vi "slow_control_alpha_01.vi"() -> ()   [LabVIEW 2018]
uses:
  <instrlib>/Lake Shore 335/Lake Shore 335.lvlib
  <instrlib>/CAEN PSM/CAEN PSM.lvlib
panel:
  in  "stop":bool
  out "Anode resets in":string
  out "Voltages":dbl[](array[numeric])
  out "Started up?":bool
  out "Try 2 Inside loop":dbl[][](array[numeric])
  in  "Read T every N cycles":i32=2
  out "Time until next cycle":dbl
  in  "Time per cycle (s)":i32=2 caption="Time Target (s)"
  in  "input cluster":errorcluster
  in  "Allows tabs on \nfront panel":T1(tab)
  in  "Heater range":u16(ring) items=["Off", "Low (On)", "Medium", "High"]
  in  "Setpoint (°C)":dbl=-100.0
  in  "PID settings":T2
  in  "COM-port NI-box":refnum<visa-resource-name>
  in  "COM-port LakeShore":refnum<visa-resource-name>
  in  "ID Query":bool=TRUE
  in  "COM-port CAEN 1":refnum<visa-resource-name>
  in  "COM-port CAEN 2":refnum<visa-resource-name>
  in  "Sensor 2 Offset":dbl=1.0 format="%#_13g"
  in  "Sensor 2 Mult. Factor":dbl=25.0 format="%#_13g"
  in  "Sensor 1 Offset":dbl=0.44736 format="%#_13g"
  in  "Sensor 1 Mult. Factor":dbl=25.0 format="%#_13g"
  in  "Sensor 3 Offset":dbl=1.0 format="%#_13g"
  in  "Sensor 3 Mult. Factor":dbl=50.0 format="%#_13g"
  in  "Sensor 4 Offset":dbl=1.0 format="%#_13g"
  in  "Sensor 4 Mult. Factor":dbl=10.0 format="%#_13g"
  in  "Ignore Initialization Errors":bool caption="Ignore init. errors?"
  out "LakeShore status":bool
  out "NI-box status":bool
  out "CAEN 1 status":bool
  out "CAEN 2 status":bool
  out "Initialization status":bool
  in  "VSet (V)":dbl[](array[numeric])
  in  "IMax (uA)":dbl[](array[numeric])
  in  "VMax (V)":dbl[](array[numeric])
  out "Cathode":dbl(knob) scale=0.0..5000.0
  out "Anode":dbl(knob) scale=0.0..4000.0
  out "PMT 2":dbl(knob) scale=0.0..1000.0
  out "PMT 1":dbl(knob) scale=1.0..1000.0
  out "Vmon (V)":dbl[](array[numeric])
  out "IMon (uA)":dbl[](array[numeric])
  in  "Reset anode":bool
  in  "Kill every Y minutes":i32=10
  in  "Keep off for X seconds":i32=10
  out "Total cycles in Anode Reset Routine":i32
  out "Current modulated cycle number":i32
  out "VSet killed":bool
  out "VSet applied":bool
  out "Read V = 0":i32
  out "Error caen 1":errorcluster
  out "Error caen 2":errorcluster
  in  "Read V every N cycles":i16=120
  # "<- Proof of concept for New/Old T + New P"
  # "PMT 1"
  # "PMT 2"
  # "Anode"
  # "Cathode"
  # "Top gate"
  # "Bottom gate"
  # "seconds"
  # "Pressure correction settings"
  # "Connection settings"
  # "Lakeshore settings"
  # "Gain (P) (XX.X)"
  # "Reset (I) (XX.X)"
  # "Rate (D) (X.X%)"
  # "Pressure correction factors go here.\nPrecisely, offsets and multiplication factors\nin the voltages passed from the pressure-\nsensors to the NI-box."
  # "<- Change wiring"
  # "Might need to split up NI-box com port.\nPreferable to task it with measuring T\nand P seperately.\nPerhaps need to set task per single channel."
  # "Alarm indicators"
  # "CAEN 1"
  # "Data"
  # "PMT 1"
  # "PMT 1"
  # "PMT 2"
  # "PMT 2"
  # "Anode"
  # "Anode"
  # "Cathode"
  # "Cathode"
  # "Arrays from CAEN 2 go here"
  # "Top gate"
  # "Top gate"
  # "Bottom gate"
  # "Bottom gate"
  # "Settings"
  # "PMT 1"
  # "PMT 1"
  # "PMT 2"
  # "PMT 2"
  # "Anode"
  # "Anode"
  # "Cathode"
  # "Cathode"
  # "CAEN 2"
  # "Top gate"
  # "Top gate"
  # "Bottom gate"
  # "Bottom gate"
  # "PMT 1"
  # "PMT 2"
  # "Anode"
  # "Cathode"
  # "Needle gauges or other displays go here"
  # "Top gate"
  # "Bottom gate"
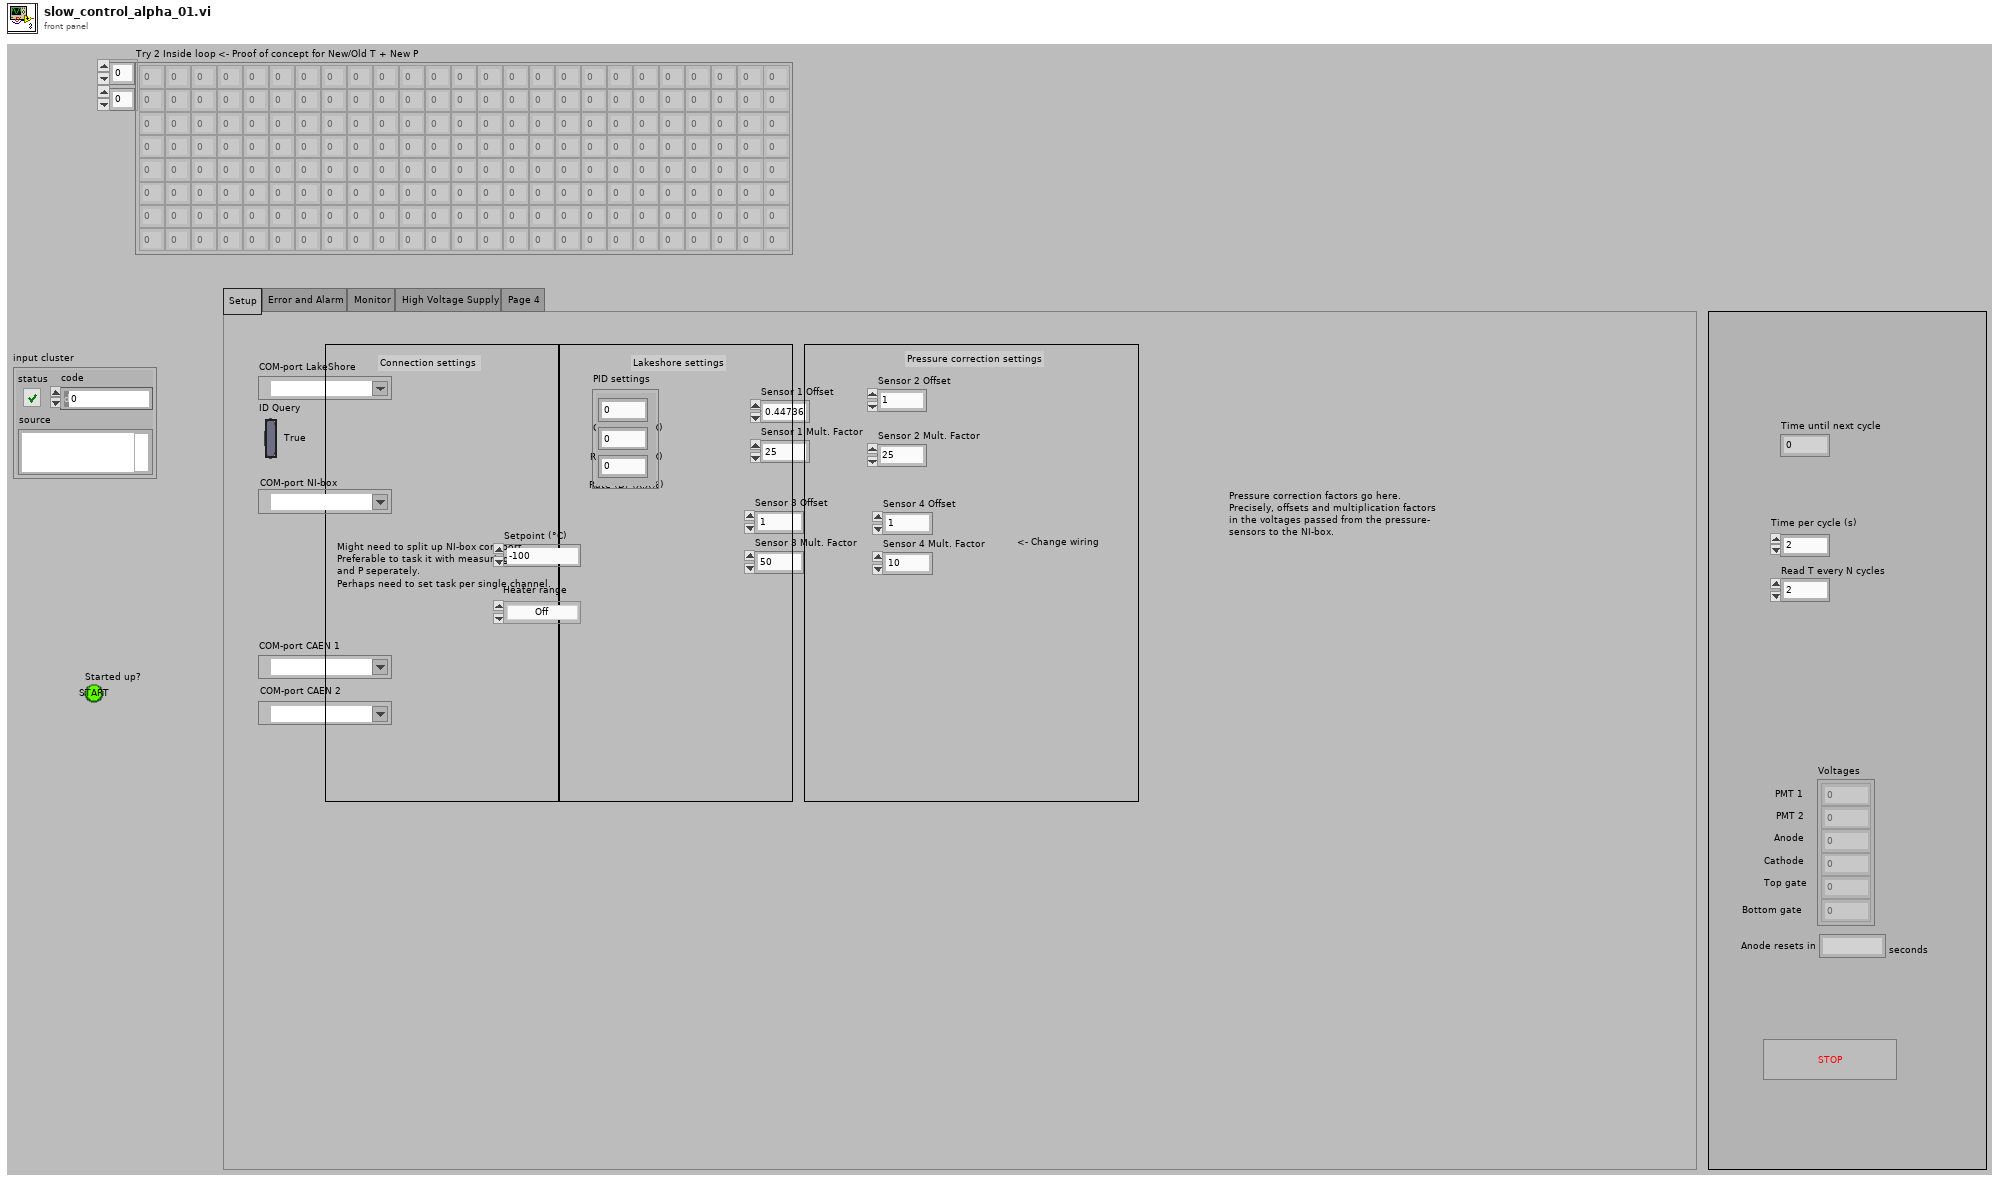
[diagram p1: front panel]
types:
  T1 = enum32{"Setup", "Error and Alarm", "Monitor", "High Voltage Supply", "Page 4"}
  T2 = cluster{"Numeric":dbl, "Numeric 2":dbl, "Numeric 3":dbl}
  T3 = cluster{"Flow Control":u16, "Stop Bits":u16, "Data Bits":u16, "Parity":u16, "Baud Rate":u32}
  T4 = cluster{"VISA resource name out":refnum<visa-resource-name>, "error out":errorcluster}
  T5 = cluster{"VMax (V)":dbl[], "IMax (uA)":dbl[], "VSet (V)":dbl[]}
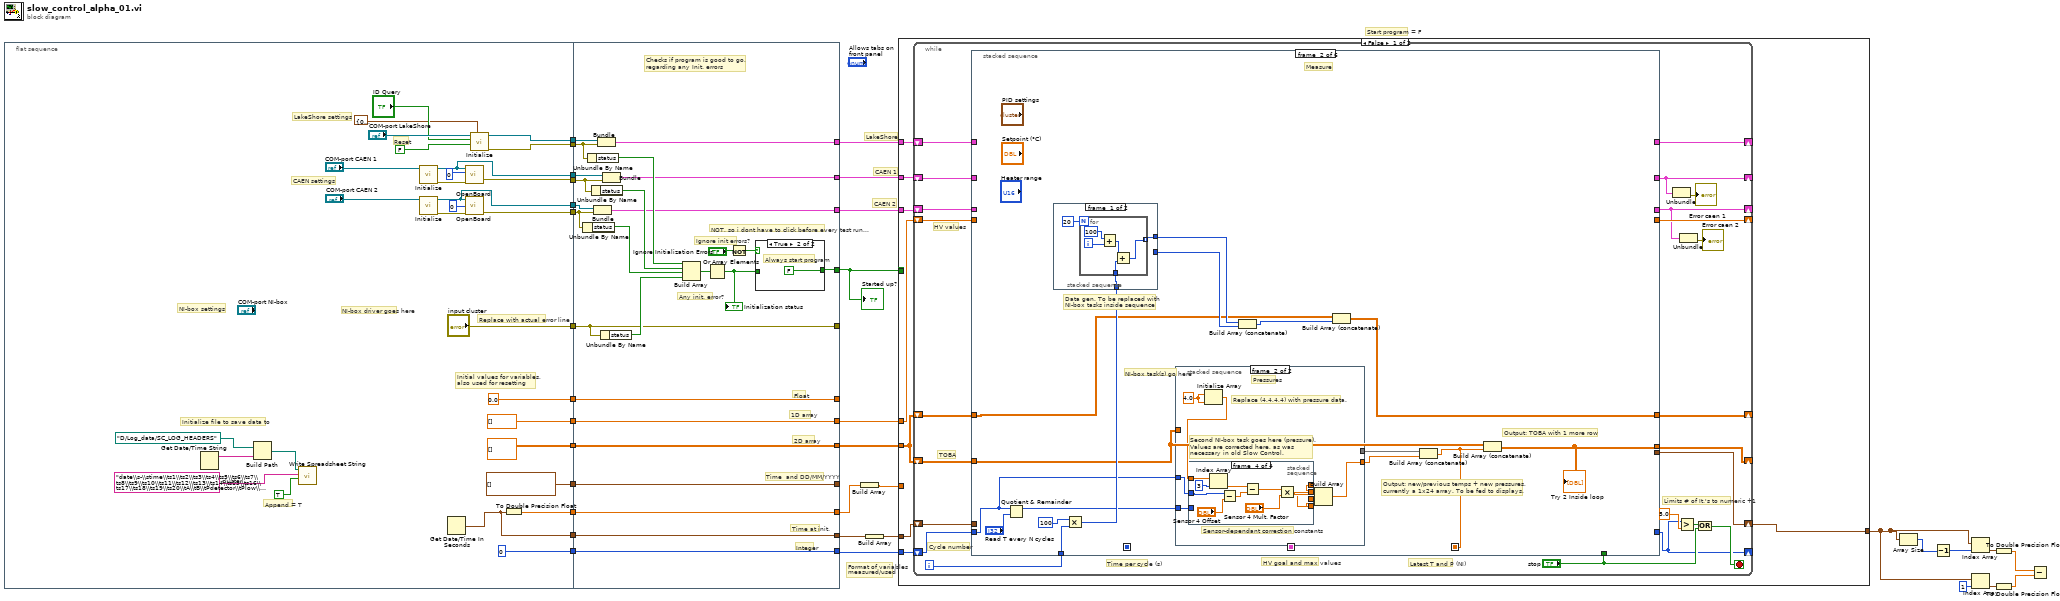
[diagram p0: block diagram]
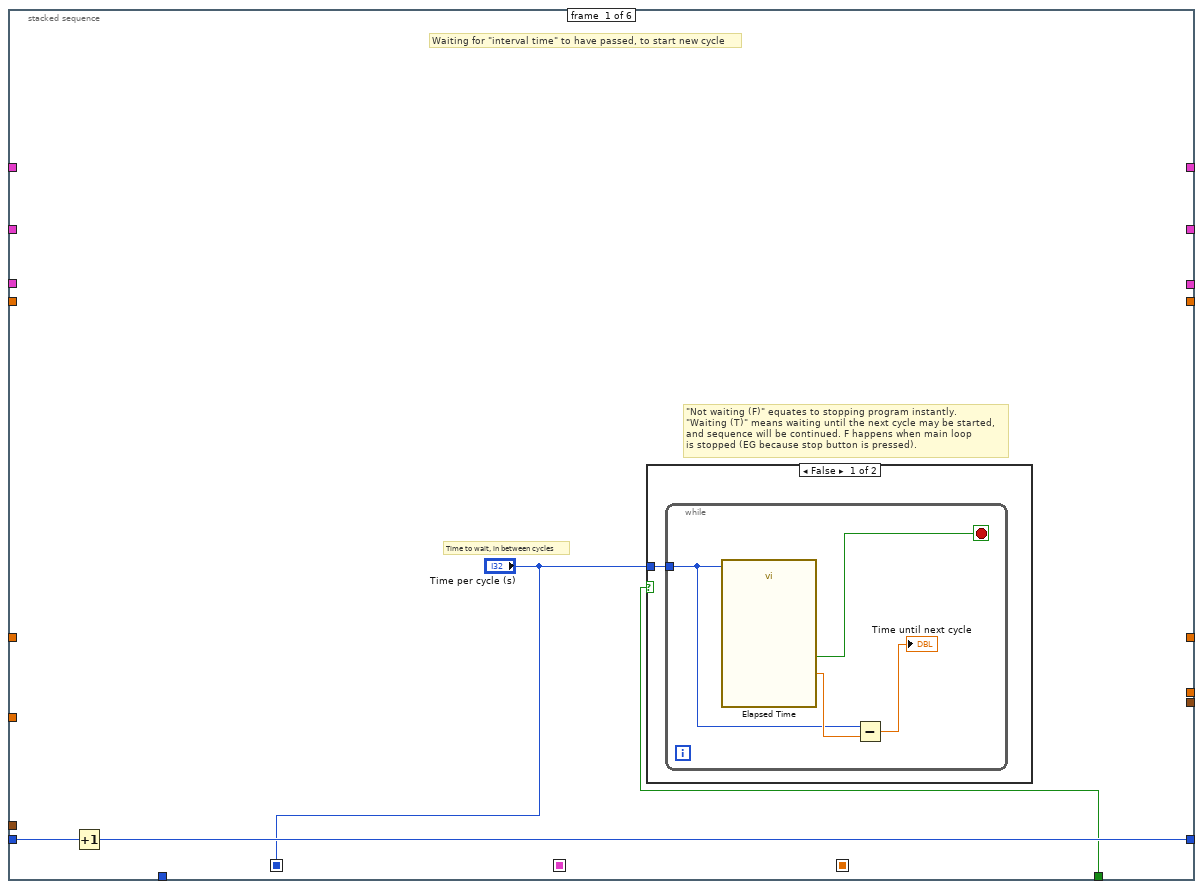
[diagram p2: hidden frame]
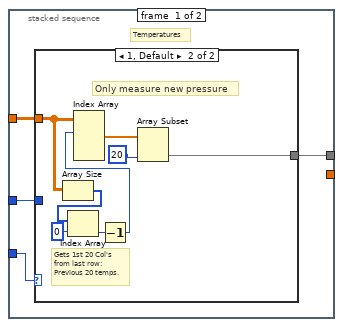
[diagram p4: hidden frame]
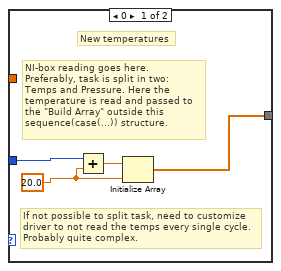
[diagram p5: hidden frame]
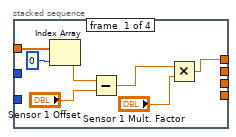
[diagram p6: hidden frame]
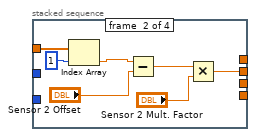
[diagram p7: hidden frame]
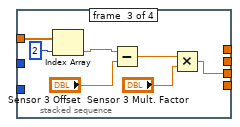
[diagram p8: hidden frame]
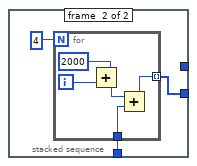
[diagram p9: hidden frame]
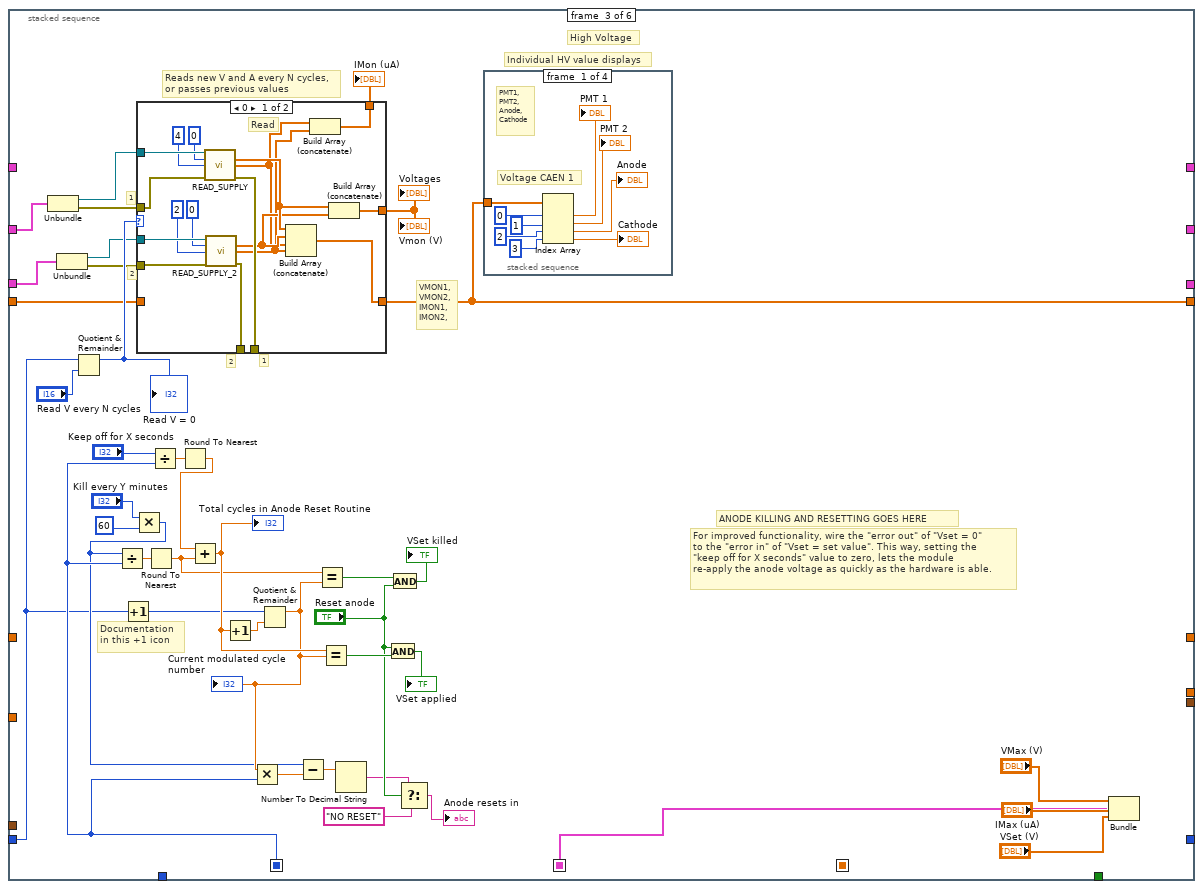
[diagram p10: hidden frame]
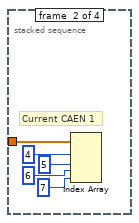
[diagram p11: hidden frame]
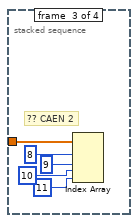
[diagram p12: hidden frame]
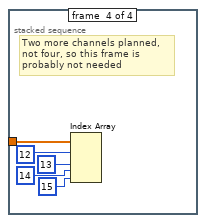
[diagram p13: hidden frame]
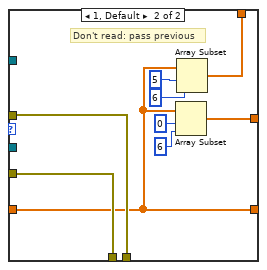
[diagram p14: hidden frame]
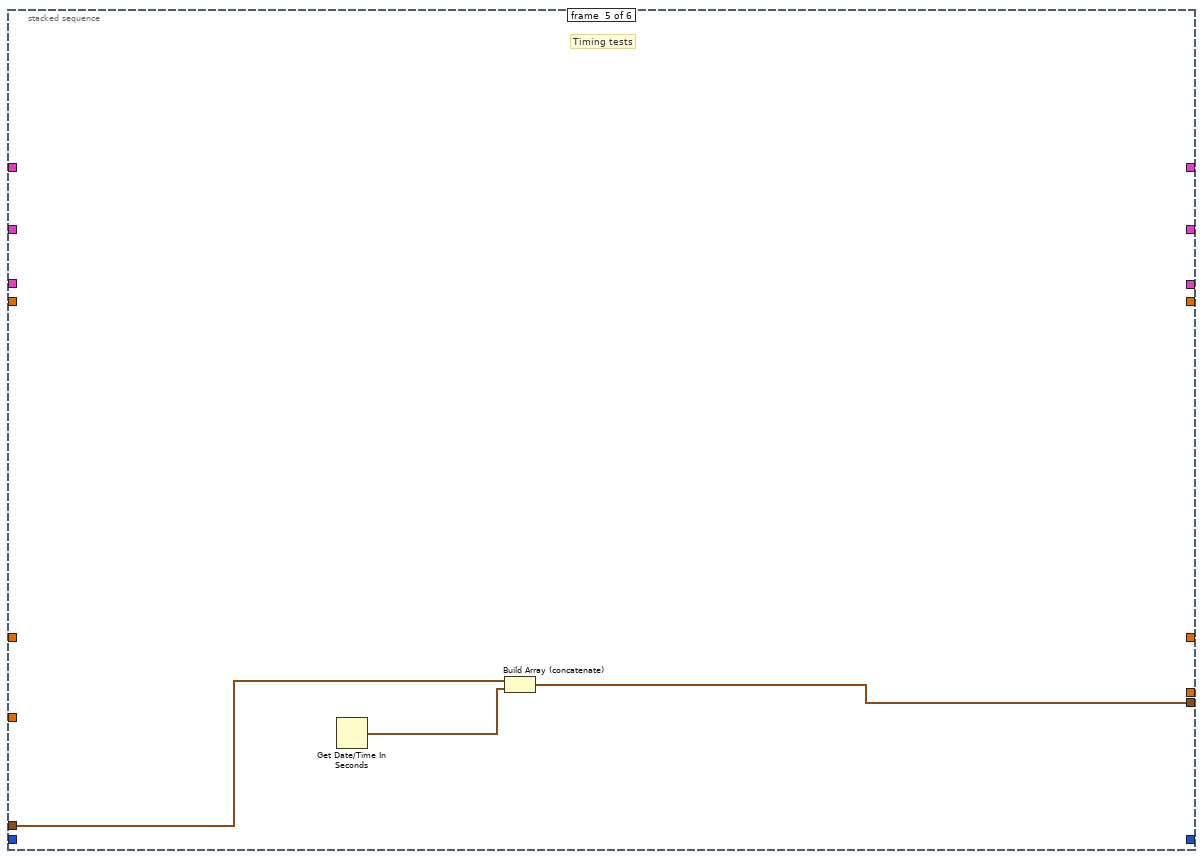
[diagram p16: hidden frame]
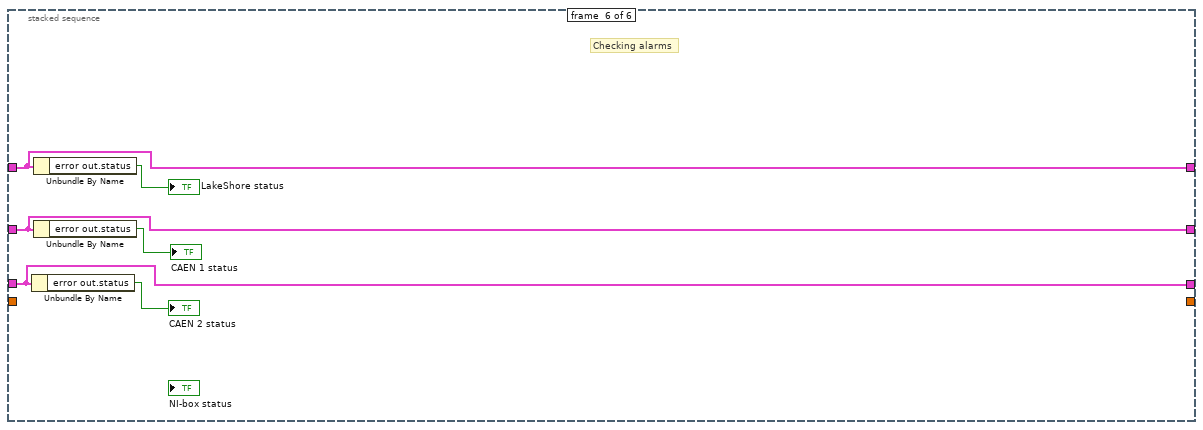
[diagram p17: hidden frame]
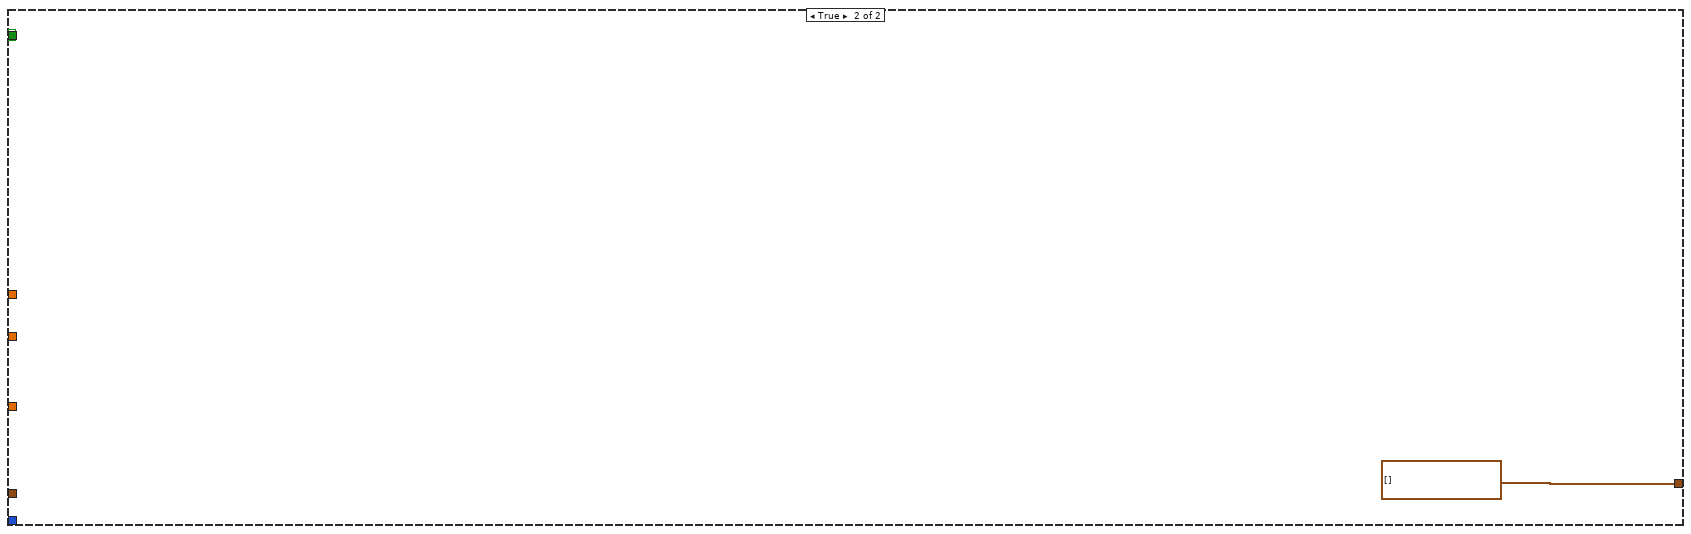
[diagram p18: hidden frame]
diagram:
  # "Start program = F"
  # "CAEN 2"
  # "CAEN 1"
  # "LakeShore"
  # "Format of variables\nmeasured/used"
  n1 = flat-sequence {
    tunnel: [w59] -> w33
    tunnel: [w58] -> w32
    tunnel: [w54] -> w31
    tunnel: [w53] -> w30
    tunnel: ["input cluster"] -> w29
    tunnel: [0.0] -> w28
    tunnel: [dbl[] []] -> w27
    tunnel: [dbl[][] []] -> w26
    tunnel: [timestamp[] []] -> w25
    tunnel: [0] -> w24
    tunnel: [w46] -> w23
    tunnel: [w39] -> w15
    tunnel: [w35] -> w4
    tunnel: [w34] -> w3
    tunnel: w33 -> [w75]
    tunnel: w32 -> [w74]
    tunnel: w31 -> [w72]
    tunnel: w30 -> [w71]
    tunnel: w29 -> [w77]
    tunnel: [w84] -> w1
    tunnel: [w82] -> _
    tunnel: w28 -> [w82]
    tunnel: [w81] -> w22
    tunnel: w27 -> [w81]
    tunnel: [w80] -> w20
    tunnel: w26 -> [w80]
    tunnel: [w79] -> _
    tunnel: w25 -> [w79]
    tunnel: [w78] -> w21
    tunnel: w24 -> [w78]
    tunnel: [w77] -> _
    tunnel: [w76] -> w17
    tunnel: w23 -> [w76]
    tunnel: [w73] -> w19
    tunnel: [w70] -> w18
    tunnel: [w67] -> w14
    tunnel: w15 -> [w67]
    tunnel: w4 -> [w65]
    tunnel: w3 -> [w64]
    tunnel: [w63] -> w2
    frame #0 {
      # "Append = T"
      # "Change to fit order of data in cluster"
      # "Initialize file to save data to"
      # "Initial values for variables,\nalso used for resetting"
      # "Replace with actual error line"
      # "NI-box driver goes here"
      # "NI-box settings"
      # "CAEN settings"
      # "Reset"
      # "LakeShore settings"
      n2 = Get Date/Time String() -> (date string=w42:string)  [unwired: 3 in, 1 out]
      n3 = Build Path(base path=path "D:/Log_data/SC_LOG_HEADERS", name or relative path=w42) -> (appended path=w45:path)
      n4 = call <vilib>:"Write Spreadsheet String.vi"("append to file? (new file:F)"=TRUE, "spreadsheet string"="date\\s-\\stime\\ts1\\ts2\\ts3\\ts4\\ts5\\ts6\\ts7\\ts8\\ts9\\ts10\\ts11\\ts12\\ts13\\ts14\\ts15\\ts16\\ts17\\ts18\\ts19\\ts20\\tA\\tB\\tPdetector\\tPlow\\tPhigh\\tFlow\\tHeater\\tSetpoint\\tCapacitance\\tTimestamp\\tInterval\\tLevel\\tV_PMT1\\tV_PMT2\\tV_Anode\\tV_cathode\\tI_PMT1\\tI_PMT2\\tI_Anode\\tI_cathode\\t\\r\\n", "file path (dialog if empty)"=w45) -> ()  [unwired: 7 in, 2 out]
      n5 = call <instrlib>:"Initialize.vi"("VISA resource name"="COM-port CAEN 1") -> ("error out"=w55:errorcluster, "VISA resource name out"=w54:refnum<visa-resource-name>)  [unwired: 9 in]
      n6 = call <instrlib>:"Initialize.vi"("VISA resource name"="COM-port CAEN 2") -> ("error out"=w36:errorcluster, "VISA resource name out"=w35:refnum<visa-resource-name>)  [unwired: 9 in]
      n7 = Get Date/Time In Seconds() -> (seconds since 1Jan1904=w39:timestamp)
      n8 = call <instrlib>:"OpenBoard.vi"("error in (no error)"=w55, "Board Address"=0, "VISA resource name"=w54) -> ("error out"=w53:errorcluster)  [unwired: 7 in, 1 out]
      n9 = call <instrlib>:"OpenBoard.vi"("error in (no error)"=w36, "Board Address"=u8 0, "VISA resource name"=w35) -> ("error out"=w34:errorcluster)  [unwired: 7 in, 1 out]
      n10 = call <instrlib>:"Initialize.vi"("Serial Configuration"=T3 {"Flow Control"=0, "Stop Bits"=10, "Data Bits"=7, "Parity"=1, "Baud Rate"=57600}, "Reset (True)"=FALSE ("Reset (LakeShore)"), "ID Query (True)"="ID Query", "VISA resource name"="COM-port LakeShore") -> ("error out"=w58:errorcluster, "VISA resource name out"=w59:refnum<visa-resource-name>)  [unwired: 6 in]
      n11 = To Double Precision Float(number=w39) -> (double precision float=w46:dbl)
    }
    frame #1 {
      # "NOT, so i dont have to click before every test run..."
      # "Time at init."
      # "Integer"
      # "Time  and DD/MM/YYYY"
      # "2D array"
      # "1D array"
      # "Float"
      # "Checks if program is good to go,\nregarding any Init. errors"
      # "Ignore init errors?"
      # "Any init. error?"
      n12 = Unbundle By Name(w64) -> ("status"=w66:bool)
      n13 = Unbundle By Name(w74) -> ("status"=w85:bool)
      n14 = Unbundle By Name(w71) -> ("status"=w87:bool)
      n15 = Bundle("VISA resource name out"=w65, "error out"=w64) -> (w63:T4)  [unwired: 1 in]
      n16 = Bundle("VISA resource name out"=w75, "error out"=w74) -> (w73:T4)  [unwired: 1 in]
      n17 = Unbundle By Name(w77) -> ("status"=w86:bool)
      n18 = Bundle("VISA resource name out"=w72, "error out"=w71) -> (w70:T4)  [unwired: 1 in]
      n19 = Build Array(w85, w87, w86, w66) -> (w88:bool[])
      n20 = Or Array Elements(Boolean array=w88) -> (logical OR=w83:bool)
      "Initialization status" <- w83
      n21 = Not(x="Ignore Initialization Errors") -> (.not. x?=w68:bool)
      n22 = case shown="True" w68 {
        tunnel: [w89 FALSE] -> w84
        tunnel: w83 -> [w89 _]
        frame False {
          # "Only start if no errors"
        }
        frame True {
          # "Always start program"
        }
      }
    }
  }
  n23 = Build Array(w17) -> (w16:dbl[])
  n24 = Build Array(w14) -> (w13:timestamp[])
  n25 = case shown="False" w1 {
    selector: w1 -> [_ w318]
    tunnel: [_ w318] -> _
    tunnel: w22 -> [w93 _]
    tunnel: w21 -> [w98 _]
    tunnel: w20 -> [w97 _]
    tunnel: w19 -> [w91 _]
    tunnel: w18 -> [w94 _]
    tunnel: w16 -> [_ _]
    tunnel: w13 -> [w96 _]
    tunnel: [w95 timestamp[] []] -> w9
    tunnel: w2 -> [w92 _]
    frame False {
      n26 = while {
        shift-right: [w109] -> _
        shift-left: w98 -> [w121]
        shift-right: [w115] -> _
        shift-left: w97 -> [w114]
        shift-right: [w112] -> _
        shift-left: w97 -> [w113]
        shift-right: [w110] -> w95
        shift-left: w96 -> [w111]
        shift-right: [w100] -> _
        shift-left: w94 -> [w108]
        shift-right: [w104] -> _
        shift-left: w93 -> [w107]
        shift-right: [w99] -> _
        shift-left: w92 -> [w106]
        shift-right: [w103] -> _
        shift-left: w91 -> [w105]
        i -> [w116]
        stop <- w117 stop-if-true
        # "Time per cycle (s)"
        # "Cycle number"
        # "HV goal and max values"
        # "HV values"
        # "TOBA"
        # "Latest T and P (NI)"
        # "Limits # of It.'s to numeric +1"
        n27 = stacked-sequence {
          seq-local: [_ w133 _ _ _ _] -> [_ _ _ _ _ _]
          seq-local: [_ _ w243 _ _ _] -> [_ _ _ _ _ _]
          seq-local: ["Time per cycle (s)" _ _ _ _ _] -> [_ _ w222 _ _ _]
          tunnel: [w124 _ _ _ _ _] -> w109
          tunnel: "stop" -> [w123 _ _ _ _ _]
          tunnel: w121 -> [w125 w131 w219 _ _ _]
          tunnel: w116 -> [_ w132 _ _ _ _]
          tunnel: w114 -> [_ w138 _ _ _ _]
          tunnel: [_ w142 _ _ _ _] -> w115
          tunnel: w113 -> [_ w134 _ _ _ _]
          tunnel: [_ w135 _ _ _ _] -> w112
          tunnel: w111 -> [_ _ _ _ w309 _]
          tunnel: [_ _ _ _ w308 _] -> w110
          tunnel: w108 -> [_ _ w256 _ _ w313]
          tunnel: w107 -> [_ _ w253 _ _ _]
          tunnel: w106 -> [_ _ w252 _ _ w312]
          tunnel: w105 -> [_ _ _ _ _ w311]
          tunnel: [_ _ _ _ _ w311] -> w103
          tunnel: [_ _ _ _ _ w313] -> w100
          tunnel: [_ _ _ _ _ w312] -> w99
          tunnel: [_ _ w249 _ _ _] -> w104
          frame #0 {
            # "Time to wait, in between cycles"
            # "\"Not waiting (F)\" equates to stopping program instantly.\n\"Waiting (T)\" means waiting until the next cycle may be started,\nand sequence will be continued. F happens when main loop \nis stopped (EG because stop button is pressed)."
            # "Waiting for \"interval time\" to have passed, to start new cycle"
            n28 = Increment(x=w125) -> (x+1=w124:i32)
            n29 = case shown="False" w123 {
              tunnel: "Time per cycle (s)" -> [w126 _]
              frame False {
                n30 = while {
                  tunnel: w126 -> [w128]
                  stop <- w130 stop-if-true
                  n31 = call "Elapsed Time"("Time Target (s)"=w128) -> ("Elapsed Time (s)"=w129:dbl, "Time has Elapsed"=w130:bool)  [unwired: 11 in, 6 out]
                  n32 = Subtract(x=w128, y=w129) -> (x-y=→"Time until next cycle":dbl)
                }
              }
              frame True {
              }
            }
          }
          frame #1 {
            # "Output: TOBA with 1 more row"
            # "Output: new/previous temps + new pressures,\ncurrently a 1x24 array. To be fed to displays."
            # "NI-box task(s) go here"
            # "Data gen. To be replaced with\nNI-box tasks inside sequence"
            # "Measure"
            n33 = Quotient & Remainder(x=w131, y="Read T every N cycles") -> (x-y*floor(x/y)=w139:i32)  [unwired: 1 out]
            n34 = Multiply(x=100, y=w132) -> (x*y=w145:i32)
            n35 = stacked-sequence {
              tunnel: [w203 _] -> w144
              tunnel: [_ w211] -> w143
              tunnel: w145 -> [w202 w210]
              frame #0 {
                n36 = for {
                  N: 20 -> [_]
                  tunnel: [w205] -> w203 mode=indexing
                  tunnel: w202 -> [w207]
                  i -> [w208]
                  n37 = Add(x=100, y=w208) -> (x+y=w206:i32)
                  n38 = Add(x=w206, y=w207) -> (x+y=w205:i32)
                }
              }
              frame #1 {
                n39 = for {
                  N: 4 -> [_]
                  tunnel: [w214] -> w211 mode=indexing
                  tunnel: w210 -> [w213]
                  i -> [w216]
                  n40 = Add(x=2000, y=w216) -> (x+y=w215:i32)
                  n41 = Add(x=w215, y=w213) -> (x+y=w214:i32)
                }
              }
            }
            n42 = stacked-sequence {
              tunnel: w139 -> [w150 w164]
              tunnel: [w149 _] -> w137
              tunnel: [_ w167] -> w136
              tunnel: w134 -> [w148 _]
              tunnel: w131 -> [w147 w163]
              frame #0 {
                # "Temperatures"
                n43 = case shown="1, Default" w150 {
                  tunnel: w148 -> [_ w159]
                  tunnel: [w152 w155] -> w149
                  tunnel: w147 -> [w151 _]
                  frame 0 {
                    w153 = 20.0 ("element")
                    # "If not possible to split task, need to customize\ndriver to not read the temps every single cycle.\nProbably quite complex."
                    # "NI-box reading goes here.\nPreferably, task is split in two: \nTemps and Pressure. Here the \ntemperature is read and passed to \nthe \"Build Array\" outside this \nsequence(case(...)) structure."
                    # "New temperatures"
                    n44 = Add(x=w151, y=w153) -> (x+y=w154:dbl)
                    n45 = Initialize Array(w154, w153) -> (w152:dbl[])
                  }
                  frame 1, Default {
                    # "Gets 1st 20 Col's\nfrom last row:\nPrevious 20 temps."
                    # "Only measure new pressure"
                    n46 = Array Size(array=w159) -> (size(s)=w161:i32[])
                    n47 = Index Array(array=w161, index=0) -> (element=w162:i32)
                    n48 = Decrement(x=w162) -> (x-1=w158:i32)
                    n49 = Index Array(array=w159, index (row) #1=w158) -> (element #1=w157:dbl[])  [unwired: 3 in, 1 out]
                    n50 = Array Subset(array=w157, length=20) -> (w155:dbl[])  [unwired: 1 in]
                  }
                }
              }
              frame #1 {
                w166 = 4.0 ("element")
                # "Replace (4,4,4,4) with pressure data."
                # "Second NI-box task goes here (pressure).\nValues are corrected here, as was \nnecessary in old Slow Control."
                # "Sensor-dependant correction constants"
                # "Pressures"
                n51 = Initialize Array(w166, w166) -> (w165:dbl[])
                n52 = stacked-sequence {
                  tunnel: w165 -> [w173 w185 w192 w201]
                  tunnel: [w174 _ _ _] -> w171
                  tunnel: [_ w180 _ _] -> w170
                  tunnel: [_ _ w187 _] -> w169
                  tunnel: [_ _ _ w197] -> w168
                  tunnel: w164 -> [_ _ _ _]
                  tunnel: w163 -> [_ _ _ w193]
                  frame #0 {
                    n53 = Index Array(array=w173, index=0) -> (element=w172:dbl)
                    n54 = Subtract(x=w172, y="Sensor 1 Offset") -> (x-y=w176:dbl)
                    n55 = Multiply(x=w176, y="Sensor 1 Mult. Factor") -> (x*y=w174:dbl)
                  }
                  frame #1 {
                    n56 = Index Array(array=w185, index=1) -> (element=w179:dbl)
                    n57 = Subtract(x=w179, y="Sensor 2 Offset") -> (x-y=w182:dbl)
                    n58 = Multiply(x=w182, y="Sensor 2 Mult. Factor") -> (x*y=w180:dbl)
                  }
                  frame #2 {
                    n59 = Index Array(array=w192, index=2) -> (element=w186:dbl)
                    n60 = Subtract(x=w186, y="Sensor 3 Offset") -> (x-y=w189:dbl)
                    n61 = Multiply(x=w189, y="Sensor 3 Mult. Factor") -> (x*y=w187:dbl)
                  }
                  frame #3 {
                    n62 = Index Array(array=w201, index=3) -> (element=w196:dbl)
                    n63 = Subtract(x=w193, y="Sensor 4 Offset") -> (x-y=w194:dbl)
                    n64 = Subtract(x=w196, y=w194) -> (x-y=w199:dbl)
                    n65 = Multiply(x=w199, y="Sensor 4 Mult. Factor") -> (x*y=w197:dbl)
                  }
                }
                n66 = Build Array(w171, w170, w169, w168) -> (w167:dbl[])
              }
            }
            n67 = Build Array (concatenate)(w144, w143) -> (w141:i32[])
            n68 = Build Array (concatenate)(w138, w141) -> (w142:dbl[][])
            n69 = Build Array (concatenate)(w137, w136) -> (w133:dbl[])
            n70 = Build Array (concatenate)(w134, w133) -> (w135:dbl[][])
            "Try 2 Inside loop" <- w135
          }
          frame #2 {
            # "VMON1, \nVMON2,\nIMON1,\nIMON2,"
            # "For improved functionality, wire the \"error out\" of \"Vset = 0\"\nto the \"error in\" of \"Vset = set value\". This way, setting the\n\"keep off for X seconds\" value to zero, lets the module \nre-apply the anode voltage as quickly as the hardware is able."
            # "ANODE KILLING AND RESETTING GOES HERE"
            # "Documentation\nin this +1 icon"
            # "Individual HV value displays"
            # "1"
            # "2"
            # "1"
            # "2"
            # "Reads new V and A every N cycles,\nor passes previous values"
            # "High Voltage"
            n71 = Unbundle(w256) -> ("VISA resource name out"=w255:refnum<visa-resource-name>, "error out"=w254:errorcluster)
            n72 = Unbundle(w252) -> ("VISA resource name out"=w251:refnum<visa-resource-name>, "error out"=w250:errorcluster)
            n73 = Quotient & Remainder(x=w219, y="Read V every N cycles") -> (x-y*floor(x/y)=w257:i32)  [unwired: 1 out]
            "Read V = 0" <- w257
            n74 = Increment(x=w219) -> (x+1=w229:i32)
            n75 = Multiply(x="Kill every Y minutes", y=60) -> (x*y=w220:i32)
            n76 = Divide(x=w220, y=w222) -> (x/y=w232:dbl)
            n77 = case shown="0" w257 {
              tunnel: w255 -> [w298 _]
              tunnel: w254 -> [w297 w306]
              tunnel: w253 -> [_ w302]
              tunnel: w251 -> [w292 _]
              tunnel: w250 -> [w291 w307]
              tunnel: [w288 w307] -> _
              tunnel: [w294 w306] -> _
              tunnel: [w293 w302] -> w249
              tunnel: [w285 w303] -> w248
              tunnel: [w282 w299] -> w247
              frame 0 {
                # "Read"
                n78 = call "READ_SUPPLY.vi"("VISA resource name"=w298, "Board address"=u8 0, "NChannels"=u8 4, "error in (no error)"=w297) -> ("VMon values (V)"=w287:dbl[], "IMon values (uA)"=w283:dbl[], "error out"=w294:errorcluster)  [unwired: 9 in]
                n79 = call "READ_SUPPLY_2.vi"("VISA resource name"=w292, "Board address"=u8 0, "NChannels"=u8 2, "error in (no error)"=w291) -> ("VMon values (V)"=w286:dbl[], "IMon values (uA)"=w284:dbl[], "error out"=w288:errorcluster)  [unwired: 9 in]
                n80 = Build Array (concatenate)(w287, w286, w283, w284) -> (w293:dbl[])
                n81 = Build Array (concatenate)(w283, w284) -> (w282:dbl[])
                n82 = Build Array (concatenate)(w287, w286) -> (w285:dbl[])
              }
              frame 1, Default {
                # "Don't read: pass previous"
                n83 = Array Subset(array=w302, index=0, length=6) -> (w303:dbl[])
                n84 = Array Subset(array=w302, index=5, length=6) -> (w299:dbl[])
              }
            }
            "Voltages" <- w248
            "Vmon (V)" <- w248
            "IMon (uA)" <- w247
            n85 = Round To Nearest(number=w232) -> (nearest integer value=w224:dbl)
            n86 = Divide(x="Keep off for X seconds", y=w222) -> (x/y=w234:dbl)
            n87 = Round To Nearest(number=w234) -> (nearest integer value=w233:dbl)
            n88 = Add(x=w233, y=w224) -> (x+y=w230:dbl)
            "Total cycles in Anode Reset Routine" <- w230
            n89 = Increment(x=w230) -> (x+1=w238:dbl)
            n90 = Quotient & Remainder(x=w229, y=w238) -> (x-y*floor(x/y)=w223:dbl)  [unwired: 1 out]
            "Current modulated cycle number" <- w223
            n91 = Multiply(x=w223, y=w222) -> (x*y=w221:dbl)
            n92 = Subtract(x=w220, y=w221) -> (x-y=w228:dbl)
            n93 = Equal?(x=w224, y=w223) -> (x = y?=w239:bool)
            n94 = Equal?(x=w230, y=w223) -> (x = y?=w241:bool)
            n95 = Number To Decimal String(number=w228) -> (decimal integer string=w227:string)  [unwired: 1 in]
            n96 = And(x="Reset anode", y=w241) -> (x .and. y?=→"VSet applied":bool)
            n97 = And(x=w239, y="Reset anode") -> (x .and. y?=→"VSet killed":bool)
            n98 = Select(t=w227, s="Reset anode", f="NO RESET") -> (s? t:f=→"Anode resets in":string)
            n99 = stacked-sequence {
              tunnel: w249 -> [w266 w267 w272 w277]
              frame #0 {
                # "Voltage CAEN 1"
                # "PMT1,\nPMT2,\nAnode,\nCathode"
                n100 = Index Array(array=w266, index #1=0 ("index"), index #2=1 ("index"), index #3=2 ("index"), index #4=3 ("index")) -> (element #1=→"PMT 1":dbl, element #2=→"PMT 2":dbl, element #3=→"Anode":dbl, element #4=→"Cathode":dbl)
              }
              frame #1 {
                # "Current CAEN 1"
                n101 = Index Array(array=w267, index #1=4 ("index"), index #2=5 ("index"), index #3=6 ("index"), index #4=7 ("index")) -> ()  [unwired: 4 out]
              }
              frame #2 {
                # "?? CAEN 2"
                n102 = Index Array(array=w272, index #1=8 ("index"), index #2=9 ("index"), index #3=10 ("index"), index #4=11 ("index")) -> ()  [unwired: 4 out]
              }
              frame #3 {
                # "Two more channels planned, \nnot four, so this frame is\nprobably not needed"
                n103 = Index Array(array=w277, index #1=12 ("index"), index #2=13 ("index"), index #3=14 ("index"), index #4=15 ("index")) -> ()  [unwired: 4 out]
              }
            }
            n104 = Bundle("VMax (V)"="VMax (V)", "IMax (uA)"="IMax (uA)", "VSet (V)"="VSet (V)") -> (w243:T5)  [unwired: 1 in]
          }
          frame #3 {
            # "Reset anode"
          }
          frame #4 {
            # "Timing tests"
            n105 = Get Date/Time In Seconds() -> (seconds since 1Jan1904=w310:timestamp)
            n106 = Build Array (concatenate)(w309, w310) -> (w308:timestamp[])
          }
          frame #5 {
            # "Checking alarms"
            n107 = Unbundle By Name(w312) -> ("error out.status"=→"CAEN 2 status":bool)
            n108 = Unbundle By Name(w311) -> ("error out.status"=→"LakeShore status":bool)
            n109 = Unbundle By Name(w313) -> ("error out.status"=→"CAEN 1 status":bool)
          }
        }
        n110 = Unbundle(w100) -> ("error out"=→"Error caen 1":errorcluster)  [unwired: 1 out]
        n111 = Greater?(x=w109, y=5.0 ("x")) -> (0:w119:bool)
        n112 = Unbundle(w99) -> ("error out"=→"Error caen 2":errorcluster)  [unwired: 1 out]
        n113 = Or(x=w119, y="stop") -> (x .or. y?=w117:bool)
      }
    }
    frame True {
    }
  }
  n114 = Array Size(array=w9) -> (size(s)=w12:i32)
  n115 = Decrement(x=w12) -> (x-1=w11:i32)
  n116 = Index Array(array=w9, index=w11) -> (element=w10:timestamp)
  n117 = Index Array(array=w9, index=1) -> (element=w7:timestamp)
  n118 = To Double Precision Float(number=w10) -> (double precision float=w6:dbl)
  n119 = To Double Precision Float(number=w7) -> (double precision float=w5:dbl)
  n120 = Subtract(x=w6, y=w5) -> ()  [unwired: 1 out]
  "Started up?" <- w1
